vi "Low Power Mode.vi"(0 "GEA2 Reference In":refnum<k24>, 5 "Action":enum16{"Enter", "Exit"}(ring), 11 "Error In":errorcluster) -> (4 "GEA2 Reference Out":refnum<k24>, 6 "Pass/Fail?":bool, 8 "Report Text":string, 15 "Error Out":errorcluster)   [LabVIEW 2016, in "Centauro.lvlib"]
doc: "Use this VI to enter or exit low power mode."
uses:
  Projects/Centauro.lvlib
  Q:/Common/DLLs/GEA3/GeaCommunication.dll
  Common/DLLs/GEA3/GeaCommunication.dll
  Common/LabVIEW GEA2 Toolkit/LabVIEW_GEA2_Toolkit.lvlibp/type defs/Source_Destination.ctl
  Common/LabVIEW GEA2 Toolkit/LabVIEW_GEA2_Toolkit.lvlibp/type defs/ERD Read Data In.ctl
  Common/LabVIEW GEA2 Toolkit/LabVIEW_GEA2_Toolkit.lvlibp/type defs/Data Type.ctl
  Common/LabVIEW GEA2 Toolkit/LabVIEW_GEA2_Toolkit.lvlibp/type defs/ERD Write Data In.ctl
  Common/LabVIEW GEA2 Toolkit/LabVIEW_GEA2_Toolkit.lvlibp
panel:
  in  "Standalone?":bool
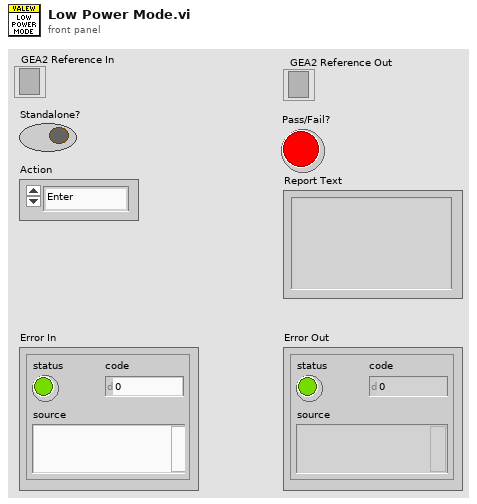
[diagram p1: front panel]
types:
  T1 = typedef "LabVIEW_GEA2_Toolkit.lvlibp/ERD Read Data In.ctl" = cluster{"ERD Number":u16, "Data Type":T2}
  T2 = typedef "LabVIEW_GEA2_Toolkit.lvlibp/Data Type.ctl" = enum16{"string", "boolean", "uint8_t", "uint16_t", "uint32_t", "uint64_t", "int8_t", "int16_t", "int32_t", "int64_t"}
  T3 = typedef "LabVIEW_GEA2_Toolkit.lvlibp/Source_Destination.ctl" = cluster{"Source":u8, "Destination":u8}
  T4 = typedef "LabVIEW_GEA2_Toolkit.lvlibp/ERD Write Data In.ctl" = cluster{"ERD Number":u16, "Data Type":T2, "Data":string}
  T5 = typedef "LabVIEW_GEA2_Toolkit.lvlibp/ERD Read Data Out.ctl" = cluster{"ERD Number":u16, "Data":string}
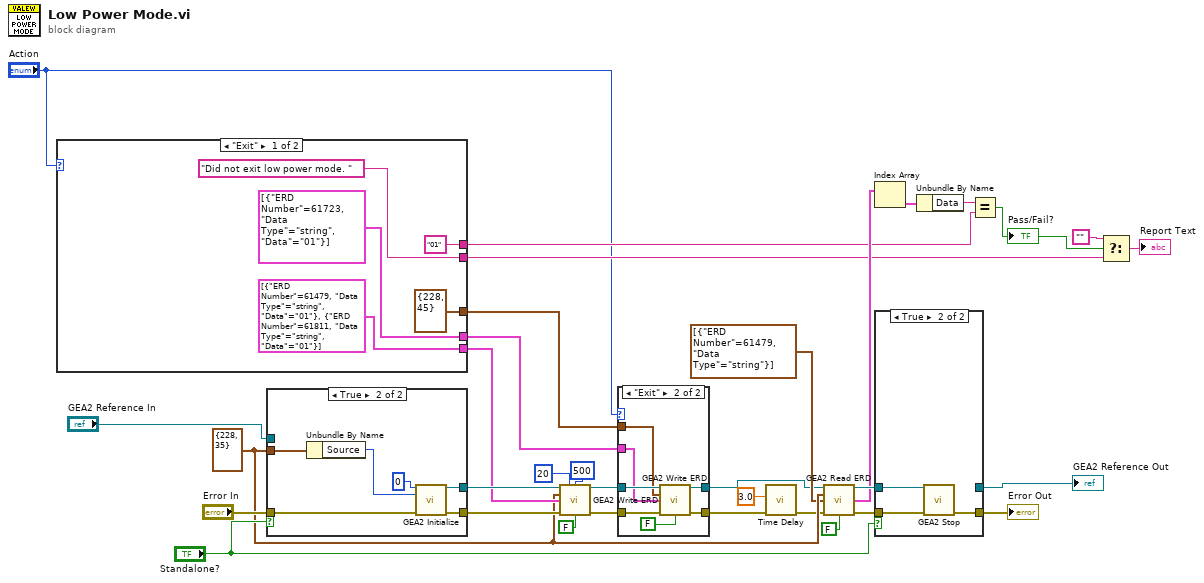
[diagram p0: block diagram]
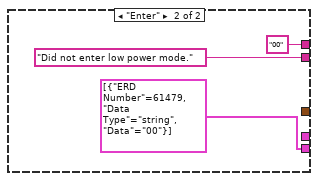
[diagram p3: hidden frame]
diagram:
  w25 = T3 {"Source"=228, "Destination"=35} ("GEA Inputs")
  n1 = case shown="\"Exit\"" "Action" {
    tunnel: [T4[] [{"ERD Number"=61479, "Data Type"=enum."string", "Data"="01"}, {"ERD Number"=61811, "Data Type"=enum."string", "Data"="01"}] ("Write ERD List") T4[] [{"ERD Number"=61479, "Data Type"=enum."string", "Data"="00"}] ("Write ERD List")] -> w26
    tunnel: ["01" ("y") "00" ("y")] -> w15
    tunnel: ["Did not exit low power mode. " ("f") "Did not enter low power mode." ("f")] -> w14
    tunnel: [T4[] [{"ERD Number"=61723, "Data Type"=enum."string", "Data"="01"}] ("Write ERD List") _] -> w5
    tunnel: [T3 {"Source"=228, "Destination"=45} ("GEA Inputs") _] -> w4
    frame "Exit" {
    }
    frame "Enter" {
    }
  }
  n2 = case shown="True" "Standalone?" {
    tunnel: "Error In" -> [w42 w49]
    tunnel: [w42 w48] -> w27
    tunnel: "GEA2 Reference In" -> [w43 _]
    tunnel: [w43 w47] -> w33
    tunnel: w25 -> [_ w45]
    frame False {
    }
    frame True {
      n3 = Unbundle By Name(w45) -> ("Source"=w46:u8)
      n4 = call "GEA2 Initialize.vi"("Board Index"=0, "Source Address"=w46, "error in"=w49) -> ("GEA2 Reference Out"=w47:refnum<k24>, "error out"=w48:errorcluster)  [unwired: 10 in, 1 out]
    }
  }
  n5 = call "GEA2 Write ERD.vi"("GEA2 Reference In"=w33, "# of Tries"=u8 20, "Read Timeout (ms)"=u32 500, "GEA Inputs"=w25, "Write ERD List"=w26, "Error In"=w27, "Verify ERD Response?"=FALSE) -> ("GEA2 Reference Out"=w8:refnum<k24>, "Error Out"=w10:errorcluster)  [unwired: 6 in, 1 out]
  n6 = case shown="\"Exit\"" "Action" {
    tunnel: [w51 w58] -> w11
    tunnel: w10 -> [w50 w57]
    tunnel: [w50 w56] -> w9
    tunnel: w8 -> [w51 w55]
    tunnel: w5 -> [_ w54]
    tunnel: w4 -> [_ w53]
    frame "Enter", Default {
    }
    frame "Exit" {
      n7 = call "GEA2 Write ERD.vi"("GEA2 Reference In"=w55, "GEA Inputs"=w53, "Write ERD List"=w54, "Error In"=w57, "Verify ERD Response?"=FALSE) -> ("GEA2 Reference Out"=w58:refnum<k24>, "Error Out"=w56:errorcluster)  [unwired: 8 in, 1 out]
    }
  }
  n8 = call "Time Delay"("error in (no error)"=w9, "Delay Time (s)"=3.0) -> ("error out"=w12:errorcluster)  [unwired: 9 in]
  n9 = call "GEA2 Read ERD.vi"("GEA2 Reference In"=w11, "GEA Inputs"=w25, "Read ERD List"=T1[] [{"ERD Number"=61479, "Data Type"=enum."string"}], "Error In"=w12, "Verify ERD Response?"=FALSE) -> ("GEA2 Reference Out"=w23:refnum<k24>, "ERD Data Out"=w19:T5[], "Error Out"=w22:errorcluster)  [unwired: 7 in, 1 out]
  n10 = Index Array(array=w19) -> (element=w18:T5)  [unwired: 1 in]
  n11 = case shown="True" "Standalone?" {
    tunnel: w22 -> [w60 w63]
    tunnel: [w60 w62] -> w32
    tunnel: [w59 _] -> w31
    tunnel: w23 -> [w59 w61]
    frame False {
    }
    frame True {
      n12 = call "GEA2 Stop.vi"("GEA2 Reference In"=w61, "Error In"=w63) -> ("Error Out"=w62:errorcluster)  [unwired: 13 in]
    }
  }
  "Error Out" <- w32
  "GEA2 Reference Out" <- w31
  n13 = Unbundle By Name(w18) -> ("Data"=w17:string)
  n14 = Equal?(x=w17, y=w15) -> (x = y?=w16:bool)
  "Pass/Fail?" <- w16
  n15 = Select(t="", s=w16, f=w14) -> (s? t:f=→"Report Text":string)
